vi "Draw 2D map.vi"(8 "error in (no error)":errorcluster, 10 "obstacles":cluster{dbl, dbl}[][](array[cluster]), 11 "bounds":T1) -> (0 "error out":errorcluster, 2 "picture":picture)   [LabVIEW 2017]
uses:
  <vilib>/Utility/miscctls.llb/LVBoundsTypeDef.ctl
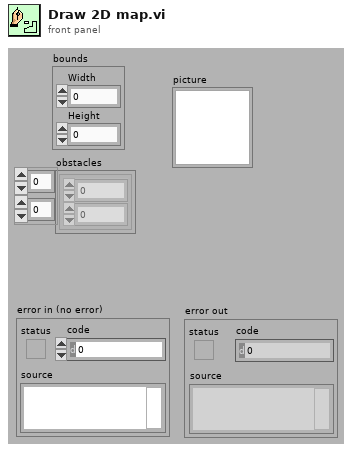
[diagram p1: front panel]
types:
  T1 = typedef "LVBoundsTypeDef.ctl" = cluster{"Width":u32, "Height":u32}
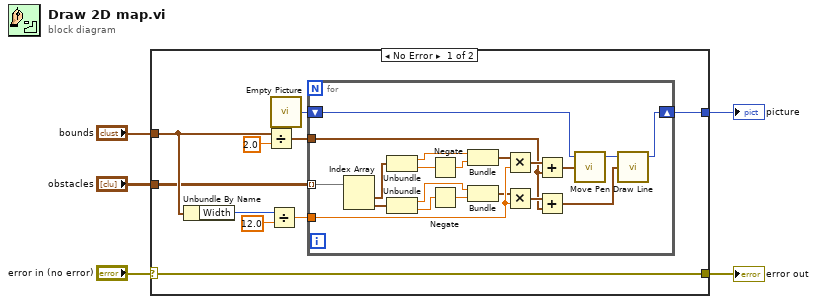
[diagram p0: block diagram]
diagram:
  n1 = case shown="No Error" "error in (no error)" {
    selector: "error in (no error)" -> [w6 w36]
    tunnel: [w15 _] -> w5
    tunnel: "bounds" -> [w12 _]
    tunnel: [w6 w36] -> w2
    tunnel: "obstacles" -> [w7 _]
    frame No Error {
      n2 = Unbundle By Name(w12) -> ("Width"=w10:u32)
      n3 = Divide(x=w12, y=2.0) -> (x/y=w14:cluster{"Width":dbl, "Height":dbl})
      n4 = Divide(x=w10, y=12.0) -> (x/y=w13:dbl)
      n5 = call "Empty Picture"() -> ("empty picture"=w8:picture)
      n6 = for {
        tunnel: w7 -> [w33] mode=indexing
        shift-right: [w28] -> w15
        shift-left: w8 -> [w35]
        tunnel: w13 -> [w30]
        tunnel: w14 -> [w31]
        n7 = Index Array(array=w33) -> (element #1=w24:cluster{dbl, dbl}, element #2=w20:cluster{dbl, dbl})  [unwired: 2 in]
        n8 = Unbundle(w24) -> (w25:dbl, w26:dbl)
        n9 = Unbundle(w20) -> (w19:dbl, w22:dbl)
        n10 = Negate(x=w26) -> (-x=w27:dbl)
        n11 = Negate(x=w22) -> (-x=w21:dbl)
        n12 = Bundle(w25, w27) -> (w23:cluster{dbl, dbl})  [unwired: 1 in]
        n13 = Bundle(w19, w21) -> (w18:cluster{dbl, dbl})  [unwired: 1 in]
        n14 = Multiply(x=w23, y=w30) -> (x*y=w32:cluster{dbl, dbl})
        n15 = Multiply(x=w18, y=w30) -> (x*y=w34:cluster{dbl, dbl})
        n16 = Add(x=w32, y=w31) -> (x+y=w16:cluster{dbl, dbl})
        n17 = Add(x=w34, y=w31) -> (x+y=w17:cluster{dbl, dbl})
        n18 = call <vilib>:"Move Pen.vi"("new position"=w16, "picture"=w35) -> ("new picture"=w29:picture)  [unwired: 3 in]
        n19 = call <vilib>:"Draw Line.vi"("picture"=w29, "end point"=w17) -> ("new picture"=w28:picture)  [unwired: 7 in]
      }
    }
    frame Error {
    }
  }
  "picture" <- w5
  "error out" <- w2
